vi "join_chat.vi"() -> (1 "username":string, 2 "ip":string, 3 "join":bool, 4 "cancel":bool)   [LabVIEW 2024]
doc: "Allows the user to write in their username and host's IP address. VI outputs a username, host's IP address and boolean values: if the user does or doesn't want to join a chat."
panel:
  in  "cancel":bool
  in  "send":bool
  in  "HOST IP ADDRESS":string
  in  "USERNAME":string
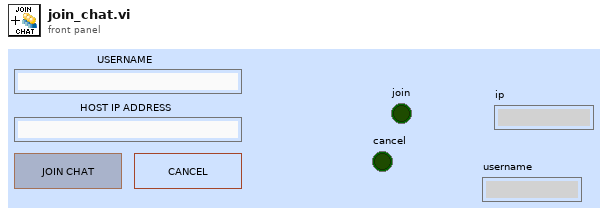
[diagram p1: front panel]
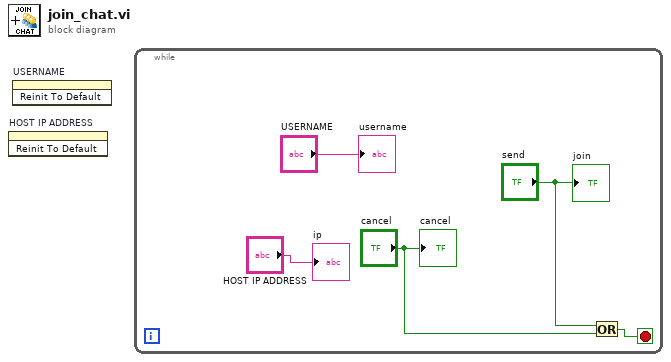
[diagram p0: block diagram]
diagram:
  n1 = invoke on="HOST IP ADDRESS" class="Str" method="Reinit To Default"() -> ()  [unwired: 3 in, 3 out]
  n2 = invoke on="USERNAME" class="Str" method="Reinit To Default"() -> ()  [unwired: 3 in, 3 out]
  n3 = while {
    stop <- w5 stop-if-true
    n4 = Or(x="send", y="cancel") -> (x .or. y?=w5:bool)
    "cancel" <- "cancel"
    "join" <- "send"
    "ip" <- "HOST IP ADDRESS"
    "username" <- "USERNAME"
  }
